vi "Main.vi"() -> ()   [LabVIEW 2025]
uses:
  <vilib>/DAQmx/read.llb/DAQmx Read (Analog 1D Wfm NChan NSamp).vi
  <vilib>/Analysis/baseanly.llb/Mean (DBL).vi
  <vilib>/DAQmx/miscellaneous.llb/DAQmx Fill In Error Info.vi
  <vilib>/Analysis/NI_AALBase.lvlib
  <vilib>/ptbypt/NI_PtbyPt.lvlib
panel:
  in  "TARE":bool
  out "Waveform Chart":waveform(dbl)[](graph)
  out "Numeric":dbl format="%.0f PSI"
  # "Autofrettage Pressure"
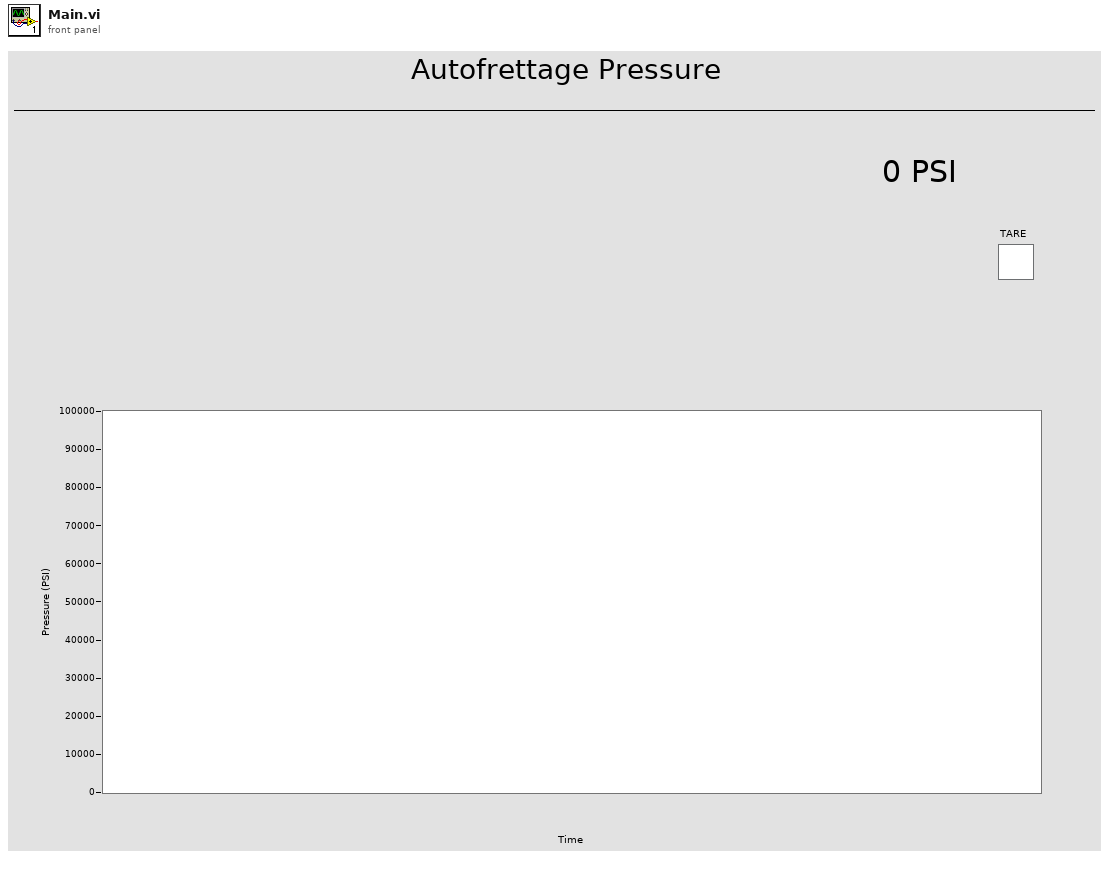
[diagram p1: front panel]
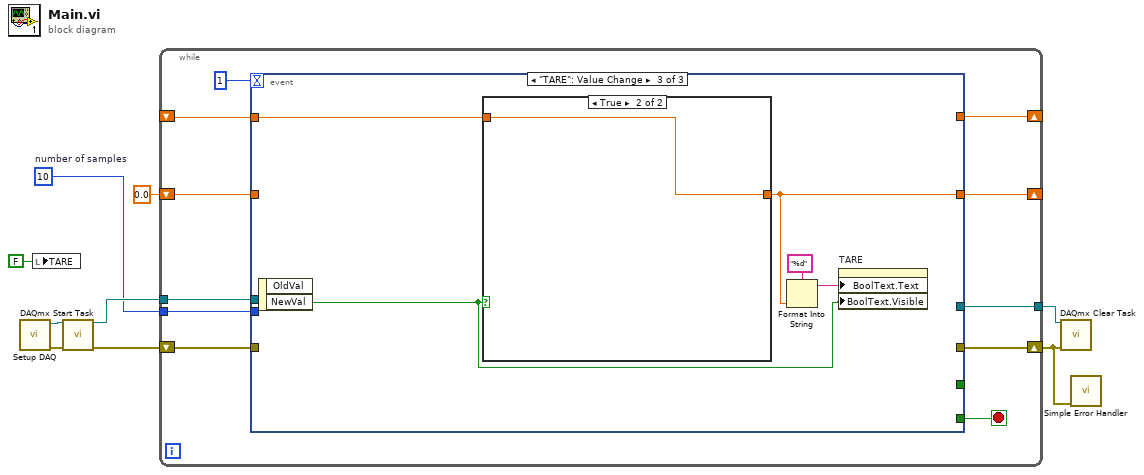
[diagram p0: block diagram]
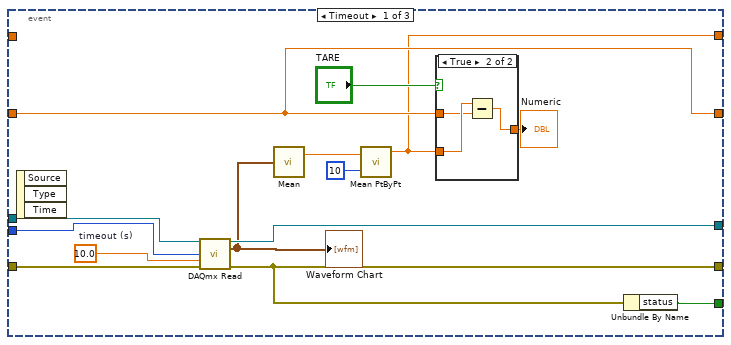
[diagram p2: hidden frame]
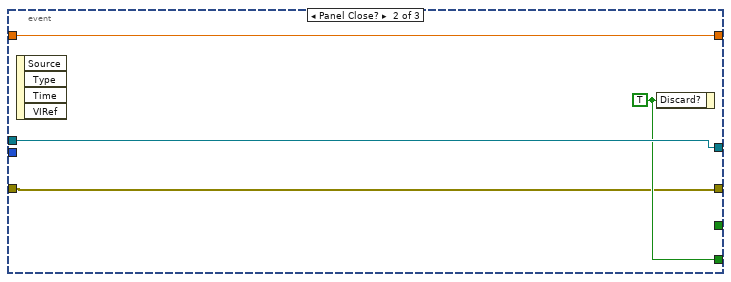
[diagram p4: hidden frame]
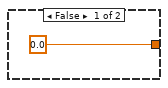
[diagram p5: hidden frame]
diagram:
  w7 = 10  # number of samples
  n1 = call "Setup DAQ.vi"() -> ("error out"=w4:errorcluster, "task out"=w5:refnum<k21>)  [unwired: 10 in]
  n2 = local write "TARE"(FALSE ("TARE")) -> ()
  n3 = call <vilib>:"DAQmx Start Task.vi"("task/channels in"=w5, "error in"=w4) -> ("task out"=w9:refnum<k21>, "error out"=w8:errorcluster)  [unwired: 12 in]
  n4 = while {
    tunnel: w9 -> [w20]
    tunnel: w7 -> [w17]
    tunnel: [w18] -> w6
    shift-right: [w16] -> w3
    shift-left: w8 -> [w19]
    shift-right: [w13] -> _
    shift-left: 0.0 -> [w12]
    shift-right: [w11] -> _
    shift-left: _ -> [w10]
    stop <- w14 stop-if-true
    n5 = event shown="[2] \"TARE\": Value Change" {
      selector: _ -> [_ _ _]
      dyn-events: _ -> [_ _ _]
      timeout: 1 -> [_ _ _]
      tunnel: w20 -> [w34 w42 _]
      tunnel: w19 -> [w33 w40 _]
      tunnel: [w32 w42 _] -> w18
      tunnel: w17 -> [w31 _ _]
      tunnel: [w30 w40 _] -> w16
      tunnel: [w27 _ _] -> _
      tunnel: [_ w41 _] -> w14
      tunnel: [w22 w39 w44] -> w13
      tunnel: w12 -> [w22 w39 _]
      tunnel: [w21 _ _] -> w11
      tunnel: w10 -> [_ _ w47]
      event Timeout {
        w29 = 10.0  # timeout (s)
        n6 = event-data() -> ()  [unwired: 1 in, 3 out]
        n7 = call-poly <vilib>:"DAQmx Read.vi"("task/channels in"=w34, "number of samples per channel"=w31, "timeout"=w29, "error in"=w33) -> ("task out"=w32:refnum<k21>, "data"=w28:waveform(dbl)[], "error out"=w30:errorcluster)  [unwired: 9 in]
        "Waveform Chart" <- w28
        n8 = call-poly <vilib>:"Mean.vi"("X"=w28) -> ("mean"=w26:dbl)  [unwired: 1 out]
        n9 = call <vilib>:"Mean PtByPt.vi"("x"=w26, "sample length"=10) -> ("mean"=w21:dbl)  [unwired: 2 in, 1 out]
        n10 = case shown="True" "TARE" {
          tunnel: w21 -> [w35 w38]
          tunnel: w22 -> [_ w37]
          tunnel: [w35 w36] -> w24
          frame False {
          }
          frame True {
            n11 = Subtract(x=w38, y=w37) -> (x-y=w36:dbl)
          }
        }
        "Numeric" <- w24
        n12 = Unbundle By Name(w30) -> ("status"=w27:bool)
      }
      event Panel Close? {
        w41 = TRUE ("Discard?")
        n13 = event-data() -> ()  [unwired: 1 in, 4 out]
        n14 = event-data("Discard?"=w41) -> ()  [unwired: 1 in, 1 out]
      }
      event "TARE": Value Change {
        n15 = event-data() -> ("NewVal"=w43:bool)  [unwired: 1 in, 1 out]
        n16 = case shown="True" w43 {
          tunnel: [0.0 ("mean") w49] -> w44
          tunnel: w47 -> [_ w49]
          frame False {
          }
          frame True {
          }
        }
        n17 = Format Into String(format string="%d", w44) -> (resulting string=w46:string)  [unwired: 2 in, 1 out]
        n18 = property on="TARE" class="Bool (strict)"("BoolText.Text"=w46, "BoolText.Visible"=w43) -> ()  [unwired: 2 in, 2 out]
      }
    }
  }
  n19 = call <vilib>:"DAQmx Clear Task.vi"("task in"=w6, "error in"=w3) -> ()  [unwired: 13 in, 1 out]
  n20 = call <vilib>:"Simple Error Handler.vi"("error in (no error)"=w3) -> ()  [unwired: 4 in, 5 out]
